vi "ManipSetShooting.vi"(3 "Parameter String":string) -> (0 "Error Out":errorcluster, 1 "Advance Trigger":bool)   [LabVIEW 2023]
doc: "This VI can switch whether the robot is shooting.\n\nParameters:\n1. \"on\" or \"off\""
uses:
  SafeParser_String.vi
  GlobalDriverStationCommands.vi
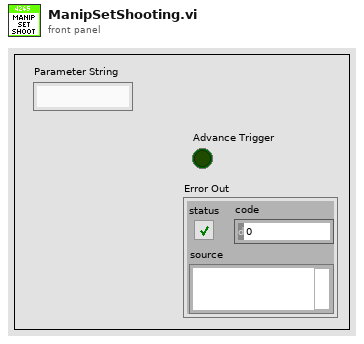
[diagram p1: front panel]
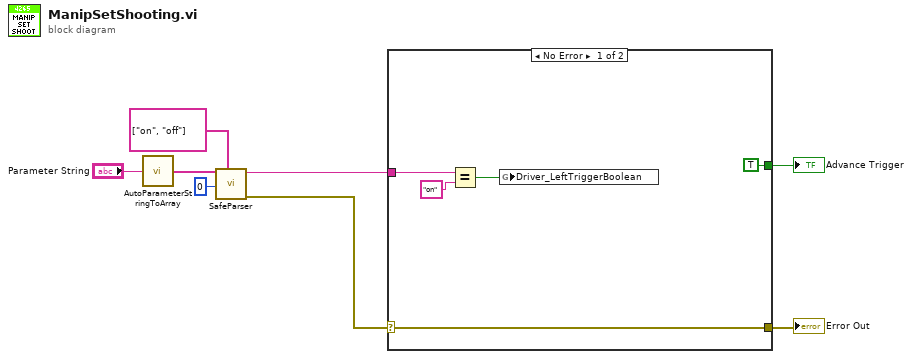
[diagram p0: block diagram]
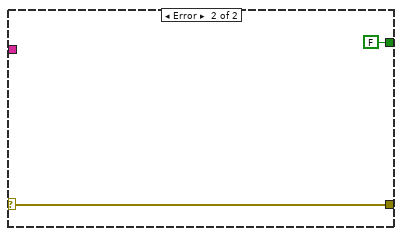
[diagram p2: hidden frame]
diagram:
  n1 = call "AutoParameterStringToArray.vi"("Parameter String"="Parameter String") -> ("Parsed Parameters"=w3:string[])
  n2 = call-poly "SafeParser.vi"("Allowed Values"=string[] ["on", "off"], "Array Index"=0 ("Parameter Index"), "String Array"=w3) -> ("Error Out"=w1:errorcluster, "Typecast Value"=w5:string)  [unwired: 7 in]
  n3 = case shown="No Error" w1 {
    selector: w1 -> [w13 w15]
    tunnel: [TRUE FALSE] -> w8
    tunnel: [w13 w15] -> w7
    tunnel: w5 -> [w12 _]
    frame No Error {
      n4 = Equal?(x=w12, y="on") -> (x = y?=w10:bool)
      n5 = global write "GlobalDriverStationCommands.vi" "Driver_LeftTriggerBoolean"(w10) -> ()
    }
    frame Error {
    }
  }
  "Advance Trigger" <- w8
  "Error Out" <- w7
